vi "graph.vi"() -> ()   [LabVIEW 2016]
panel:
  out "Waveform Graph 3":cluster{i32, i32, dbl[]}[](graph)
  out "Waveform Graph 2":dbl[][](graph)
  out "Waveform Graph 1":cluster{i32, i32, dbl[]}(graph)
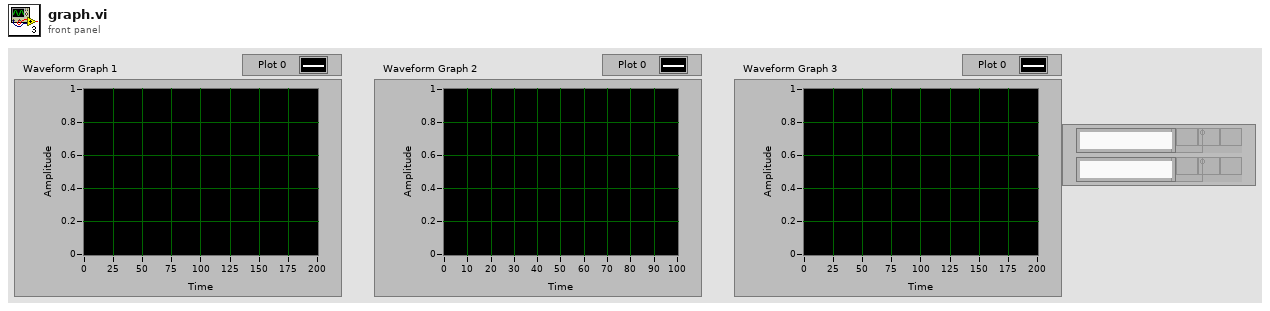
[diagram p1: front panel]
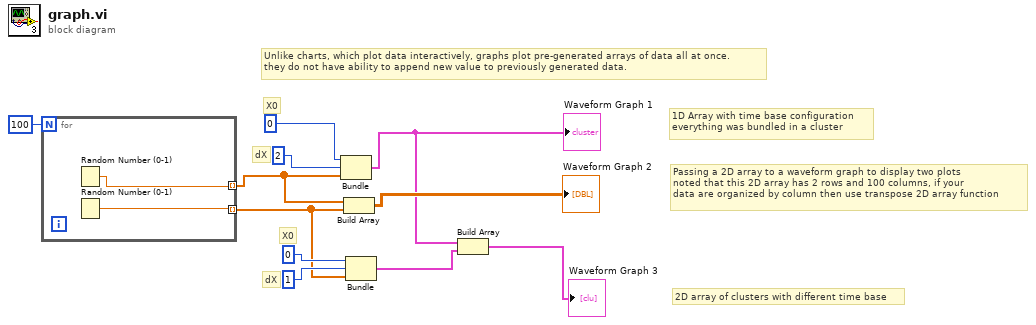
[diagram p0: block diagram]
diagram:
  # "2D array of clusters with different time base"
  # "dX"
  # "X0"
  # "Passing a 2D array to a waveform graph to display two plots\nnoted that this 2D array has 2 rows and 100 columns, if your \ndata are organized by column then use transpose 2D array function"
  # "Unlike charts, which plot data interactively, graphs plot pre-generated arrays of data all at once.\nthey do not have ability to append new value to previously generated data."
  # "1D Array with time base configuration\neverything was bundled in a cluster"
  # "dX"
  # "X0"
  n1 = for {
    N: 100 -> [_]
    tunnel: [w13] -> w8 mode=indexing
    tunnel: [w12] -> w4 mode=indexing
    n2 = Random Number (0-1)() -> (number: 0 to 1=w13:dbl)
    n3 = Random Number (0-1)() -> (number: 0 to 1=w12:dbl)
  }
  n4 = Bundle(0, 2, w8) -> (w3:cluster{i32, i32, dbl[]})  [unwired: 1 in]
  "Waveform Graph 1" <- w3
  n5 = Build Array(w8, w4) -> (→"Waveform Graph 2":dbl[][])
  n6 = Bundle(0, 1, w4) -> (w2:cluster{i32, i32, dbl[]})  [unwired: 1 in]
  n7 = Build Array(w3, w2) -> (→"Waveform Graph 3":cluster{i32, i32, dbl[]}[])
